vi "computeIncrementedString.vi"(10 "Input String":string, 11 "StringIncrement":refnum<class "StringIncrement.lvclass">) -> (2 "Incremented String":string, 3 "StringIncrement out":refnum<class "StringIncrement.lvclass">)   [LabVIEW 2013, in "UniqueName.lvlib" / "StringIncrement.lvclass"]
uses:
  StringIncrement.lvclass
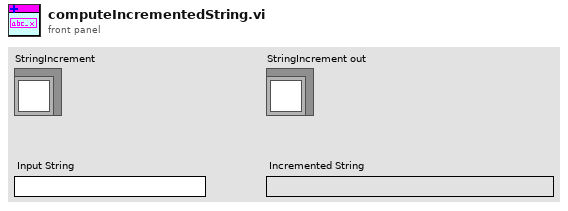
[diagram p1: front panel]
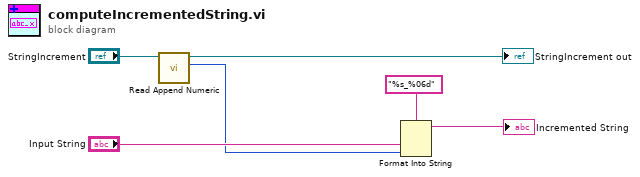
[diagram p0: block diagram]
diagram:
  n1 = call "Read Append Numeric.vi"("StringIncrement"="StringIncrement") -> ("Append Numeric"=w1:u32, "StringIncrement out"=→"StringIncrement out":refnum<class "StringIncrement.lvclass">)  [unwired: 9 in]
  n2 = Format Into String(format string="%s_%06d", "Input String", w1) -> (resulting string=→"Incremented String":string)  [unwired: 2 in, 1 out]
